vi "set_current_offset.vi"(8 "error in (no error)":errorcluster, 10 "current offset (samples)":i32, 11 "GenericWriteSignals.lvclass in":refnum<class "GenericSignalWriter.lvclass">) -> (0 "error out":errorcluster, 3 "GenericWriteSignals.lvclass out":refnum<class "GenericSignalWriter.lvclass">)   [LabVIEW 2010, in "GenericSignalWriter.lvclass"]
uses:
  GenericSignalWriter.lvclass
  GenericSignalWriter.lvclass/GenericSignalWriter.ctl
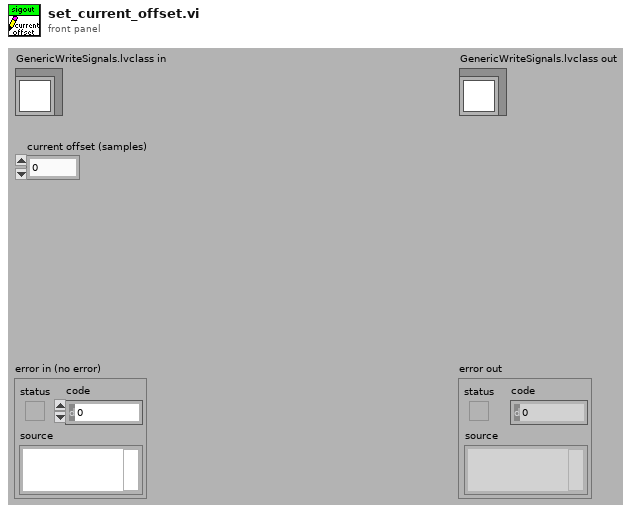
[diagram p1: front panel]
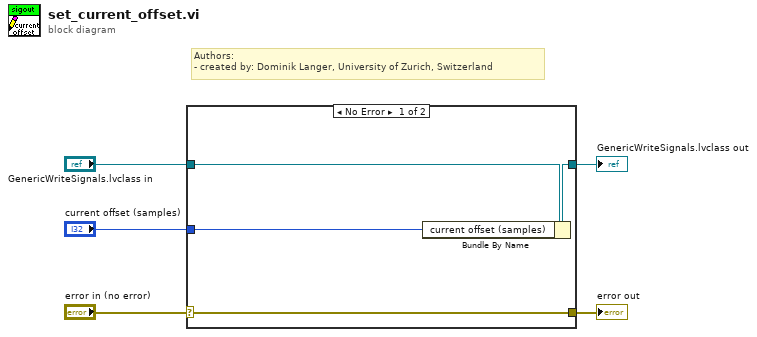
[diagram p0: block diagram]
diagram:
  # "Authors: \n- created by: Dominik Langer, University of Zurich, Switzerland"
  n1 = case shown="No Error" "error in (no error)" {
    selector: "error in (no error)" -> [w9 w10]
    tunnel: [w9 w10] -> w4
    tunnel: [w7 w11] -> w2
    tunnel: "GenericWriteSignals.lvclass in" -> [w8 w11]
    tunnel: "current offset (samples)" -> [w6 _]
    frame No Error {
      n2 = Bundle By Name(cluster=w8, "current offset (samples)"=w6) -> (w7:refnum<class "GenericSignalWriter.lvclass">)
    }
    frame Error {
    }
  }
  "error out" <- w4
  "GenericWriteSignals.lvclass out" <- w2
